vi "Load.vi"(8 "error in":errorcluster, 10 "Source":string="D:\\git\\HAL\\Source\\Tests\\resources\\instruments.xlsx", 11 "Config from EXCEL in":refnum<class "Config from EXCEL.lvclass">) -> (0 "error out":errorcluster, 3 "Config from EXCEL out":refnum<class "Config from EXCEL.lvclass">)   [LabVIEW 2025, in "Config from EXCEL.lvclass"]
uses:
  Config from EXCEL.lvclass
  Config from EXCEL.lvclass/Config from EXCEL.ctl
  Open-Xml-LabVIEW/Source/Open Xml.lvlib
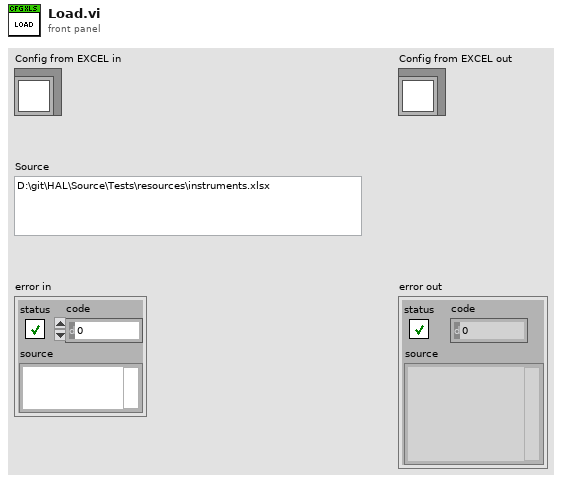
[diagram p1: front panel]
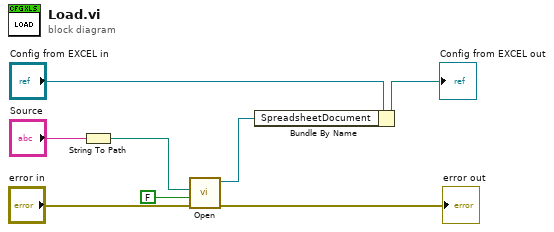
[diagram p0: block diagram]
diagram:
  n1 = String To Path(string="Source") -> (path=w1:path)
  n2 = call "Open.vi"("error in"="error in", "isEditable"=FALSE, "Path"=w1) -> ("error out"=→"error out":errorcluster, "SpreadsheetDoc"=w2:refnum<k24>)  [unwired: 7 in]
  n3 = Bundle By Name(cluster="Config from EXCEL in", "SpreadsheetDocument"=w2) -> (→"Config from EXCEL out":refnum<class "Config from EXCEL.lvclass">)
